vi "Untitled 6 (SubVI).vi"(6 "Angle Y":dbl format="%0.2f", 9 "Angle Z":dbl format="%0.2f", 10 "Angle X":dbl format="%0.2f", 11 "SceneObject in":refnum<vi>) -> (3 "SceneObject out":refnum<vi>)   [LabVIEW 2020]
uses:
  <vilib>/picture/3D Picture Control/NI_3D Picture Control.lvlib
  <vilib>/Analysis/NI_AALPro.lvlib
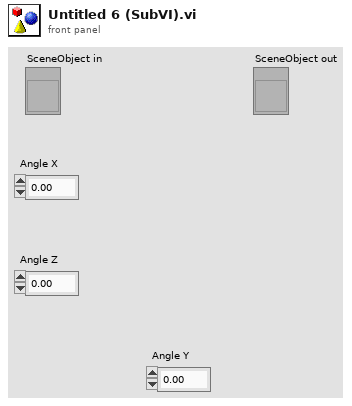
[diagram p1: front panel]
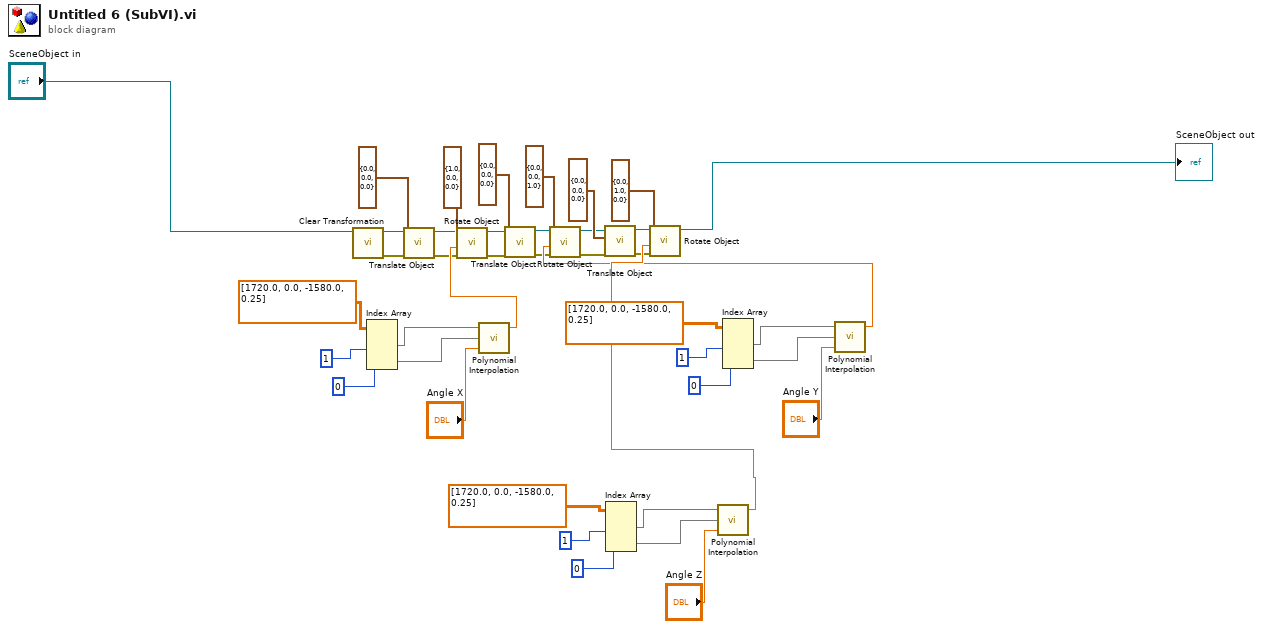
[diagram p0: block diagram]
diagram:
  n1 = call <vilib>:"Clear Transformation.vi"("Object Refnum In"="SceneObject in") -> ("error out"=w6:errorcluster, "Object Refnum Out"=w2:refnum<vi>)  [unwired: 9 in]
  n2 = Index Array(array=dbl[][] [[1720.0, 0.0], [-1580.0, 0.25]], index (col) #1=1 ("disabled index (col)"), index (col) #2=0 ("index (col)")) -> (element #1=w13:dbl[], element #2=w14:dbl[])  [unwired: 2 in]
  n3 = call <vilib>:"Translate Object.vi"("error in (no error)"=w6, "Translation"=cluster{"X":sgl, "Y":sgl, "Z":sgl} {"X"=0.0, "Y"=0.0, "Z"=0.0}, "Scene.Object In"=w2) -> ("error out"=w7:errorcluster, "Scene.Object Out"=w3:refnum<vi>)  [unwired: 7 in]
  n4 = call <vilib>:"Polynomial Interpolation.vi"("x value"="Angle X", "X"=w14, "Y"=w13) -> ("interpolation value"=w22:dbl)  [unwired: 2 out]
  n5 = call <vilib>:"Rotate Object.vi"("error in (no error)"=w7, "Angle"=w22, "Axis"=cluster{"X":sgl, "Y":sgl, "Z":sgl} {"X"=1.0, "Y"=0.0, "Z"=0.0}, "Scene.Object In"=w3) -> ("error out"=w8:errorcluster, "Scene.Object Out"=w4:refnum<vi>)  [unwired: 6 in]
  n6 = call <vilib>:"Translate Object.vi"("error in (no error)"=w8, "Translation"=cluster{"X":sgl, "Y":sgl, "Z":sgl} {"X"=0.0, "Y"=0.0, "Z"=0.0}, "Scene.Object In"=w4) -> ("error out"=w9:errorcluster, "Scene.Object Out"=w5:refnum<vi>)  [unwired: 7 in]
  n7 = Index Array(array=dbl[][] [[1720.0, 0.0], [-1580.0, 0.25]], index (col) #1=1 ("disabled index (col)"), index (col) #2=0 ("index (col)")) -> (element #1=w35:dbl[], element #2=w36:dbl[])  [unwired: 2 in]
  n8 = call <vilib>:"Polynomial Interpolation.vi"("x value"="Angle Z", "X"=w36, "Y"=w35) -> ("interpolation value"=w38:dbl)  [unwired: 2 out]
  n9 = Index Array(array=dbl[][] [[1720.0, 0.0], [-1580.0, 0.25]], index (col) #1=1 ("disabled index (col)"), index (col) #2=0 ("index (col)")) -> (element #1=w19:dbl[], element #2=w20:dbl[])  [unwired: 2 in]
  n10 = call <vilib>:"Polynomial Interpolation.vi"("x value"="Angle Y", "X"=w20, "Y"=w19) -> ("interpolation value"=w23:dbl)  [unwired: 2 out]
  n11 = call <vilib>:"Rotate Object.vi"("error in (no error)"=w9, "Angle"=w23, "Axis"=cluster{"X":sgl, "Y":sgl, "Z":sgl} {"X"=0.0, "Y"=0.0, "Z"=1.0}, "Scene.Object In"=w5) -> ("error out"=w30:errorcluster, "Scene.Object Out"=w29:refnum<vi>)  [unwired: 6 in]
  n12 = call <vilib>:"Translate Object.vi"("error in (no error)"=w30, "Translation"=cluster{"X":sgl, "Y":sgl, "Z":sgl} {"X"=0.0, "Y"=0.0, "Z"=0.0}, "Scene.Object In"=w29) -> ("error out"=w28:errorcluster, "Scene.Object Out"=w27:refnum<vi>)  [unwired: 7 in]
  n13 = call <vilib>:"Rotate Object.vi"("error in (no error)"=w28, "Angle"=w38, "Axis"=cluster{"X":sgl, "Y":sgl, "Z":sgl} {"X"=0.0, "Y"=1.0, "Z"=0.0}, "Scene.Object In"=w27) -> ("Scene.Object Out"=→"SceneObject out":refnum<vi>)  [unwired: 6 in, 1 out]
